vi "BurnIn Timer.vi"(9 "Msg":string, 10 "Time Target (s)":dbl=1.0) -> (2 "Time has Elapsed":bool)   [LabVIEW 2023]
panel:
  out "Hours":i32
  out "Minutes":i32
  out "Seconds":i32
  out "Numeric":u16
  in  "stop":bool
  out "error out":errorcluster
  out "Get Start Time (s)":dbl
  out "Present (s)":dbl
  out "Elapsed Time (s)":dbl
  in  "Auto Reset":bool=TRUE
  in  "error in (no error)":errorcluster
  in  "Set Start Time (s)":dbl
  in  "Reset":bool
  # ":"
  # ":"
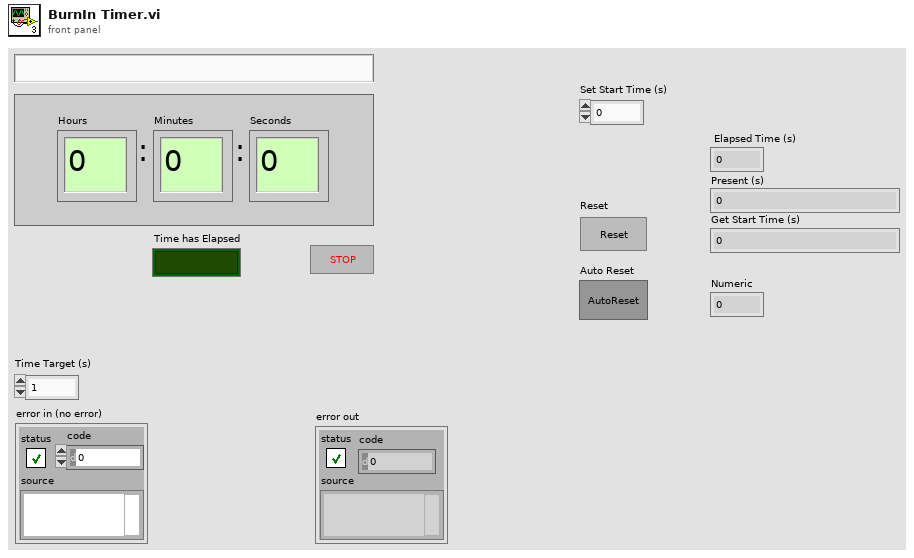
[diagram p1: front panel]
types:
  T1 = typedef "LVDateTimeRec.ctl" = cluster{"fractional second":dbl, "second":i32, "minute":i32, "hour":i32, "day of month":i32, "month":i32, "year":i32, "day of week":i32, "day of year":i32, "DST":i32}
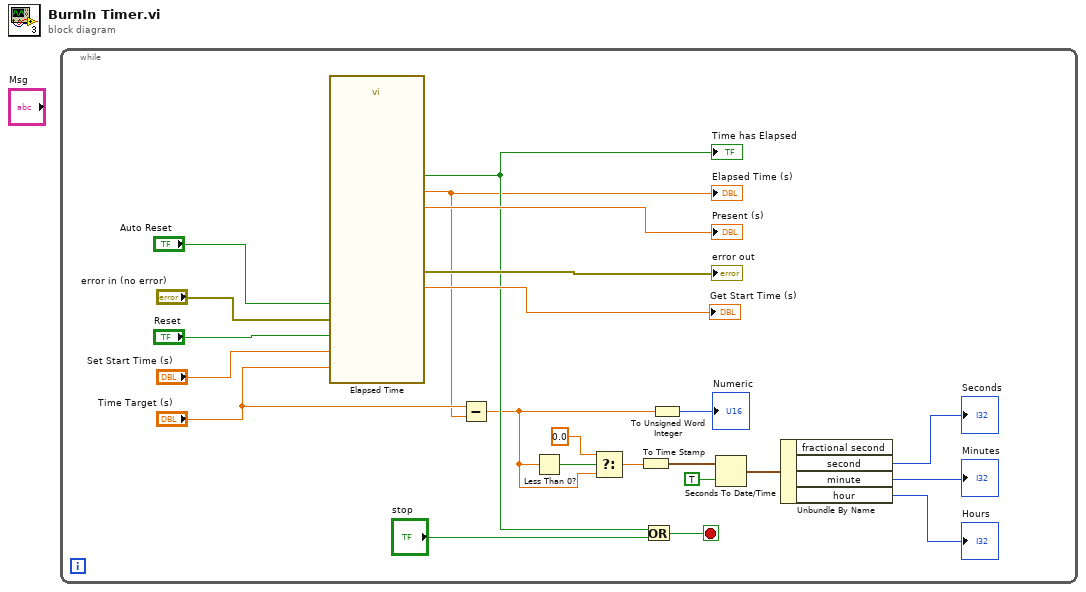
[diagram p0: block diagram]
diagram:
  n1 = while {
    stop <- w14 stop-if-true
    n2 = call "Elapsed Time"("Time Target (s)"="Time Target (s)", "Reset"="Reset", "Auto Reset"="Auto Reset", "error in (no error)"="error in (no error)", "Set Start Time (s)"="Set Start Time (s)") -> ("Get Start Time (s)"=→"Get Start Time (s)":dbl, "Present (s)"=→"Present (s)":dbl, "Elapsed Time (s)"=w12:dbl, "Time has Elapsed"=w15:bool, "error out"=→"error out":errorcluster)  [unwired: 7 in, 3 out]
    "Time has Elapsed" <- w15
    "Elapsed Time (s)" <- w12
    n3 = Subtract(x="Time Target (s)", y=w12) -> (x-y=w5:dbl)
    n4 = Less Than 0?(x=w5) -> (x < 0?=w7:bool)
    n5 = Select(t=0.0, s=w7, f=w5) -> (s? t:f=w4:dbl)
    n6 = To Time Stamp(1:w4) -> (0:w8:timestamp)
    n7 = Or(x=w15, y="stop") -> (x .or. y?=w14:bool)
    n8 = To Unsigned Word Integer(number=w5) -> (unsigned 16bit integer=→"Numeric":u16)
    n9 = Seconds To Date/Time(time stamp (now)=w8, to UTC (F)=TRUE) -> (date time rec=w9:T1)
    n10 = Unbundle By Name(w9) -> ("second"=→"Seconds":i32, "minute"=→"Minutes":i32, "hour"=→"Hours":i32)  [unwired: 1 out]
  }
